vi "test_Multiple Writes and Reads.vi"(8 "error in (no error)":errorcluster, 11 "Scalar Channels Testing in":refnum<class "FPGA Addon Scalar Channels System Tests.lvclass">) -> (0 "error out":errorcluster, 3 "Scalar Channels Testing out":refnum<class "FPGA Addon Scalar Channels System Tests.lvclass">)   [LabVIEW 2018, in "FPGA Addon Scalar Channels System Tests.lvclass"]
uses:
  FPGA Addon Scalar Channels System Tests.lvclass
  C:/Dev/niveristand-fpga-addon-custom-device-1/Source/Tests/FPGA Addon Test Class/FPGA Addon Test Class.lvclass
  C:/Program Files (x86)/National Instruments/LabVIEW 2018/vi.lib/NI/NI VS CD Testing Tools/VeriStandTestCase/VeriStandTestCase.lvclass
  FPGA Addon Test Class/FPGA Addon Test Class.lvclass/FPGA Addon Test Class.ctl
  FPGA Addon Test Class/FPGA Addon Test Class.lvclass
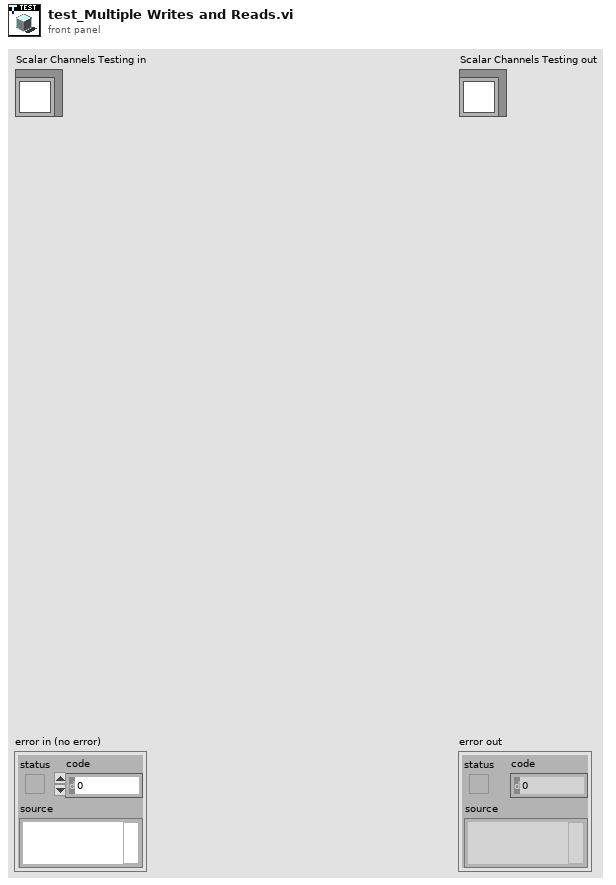
[diagram p1: front panel]
types:
  T1 = typedef "NI_VS Workspace ExecutionAPI.lvlib/WorkspaceAPI.ctl" = refnum<k24>
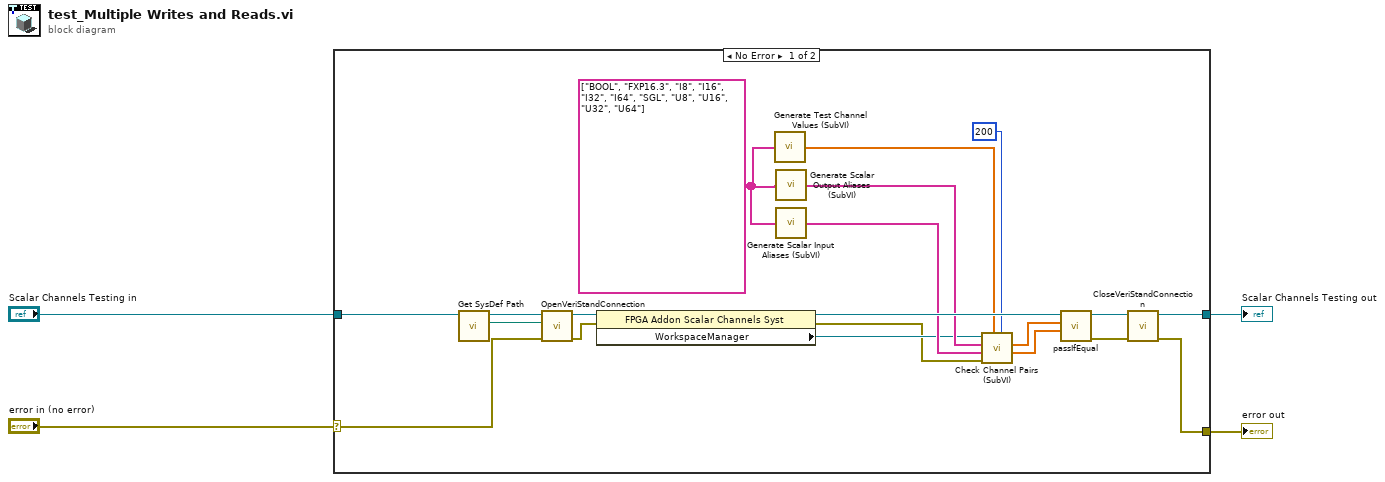
[diagram p0: block diagram]
diagram:
  n1 = case shown="No Error" "error in (no error)" {
    selector: "error in (no error)" -> [w17 w26]
    tunnel: [w23 w26] -> w3
    tunnel: [w24 w25] -> w1
    tunnel: "Scalar Channels Testing in" -> [w7 w25]
    frame No Error {
      w12 = string[] ["BOOL", "FXP16.3", "I8", "I16", "I32", "I64", "SGL", "U8", "U16", "U32", "U64"]
      n2 = call "Get SysDef Path.vi"("Scalar Channels Testing in"=w7) -> ("SysDef Path"=w5:path, "Scalar Channels Testing out"=w6:refnum<class "FPGA Addon Scalar Channels System Tests.lvclass">)  [unwired: 9 in]
      n3 = call-dynamic "OpenVeriStandConnection.vi"("error in (no error)"=w17, "System Definition File"=w5, "VeriStand Test Case in"=w6) -> ("error out"=w22:errorcluster, "VeriStand Test Case out"=w21:refnum<class "FPGA Addon Scalar Channels System Tests.lvclass">)  [unwired: 6 in, 1 out]
      n4 = property class="FPGA Addon Scalar Channels Syst"(reference=w21, error in=w22) -> (reference out=w19:refnum<class "FPGA Addon Scalar Channels System Tests.lvclass">, error out=w8:errorcluster, "WorkspaceManager"=w9:T1)
      n5 = call "Generate Test Channel Values (SubVI).vi"("Aliases in"=w12) -> ("Test Channel Values out"=w14:dbl[])
      n6 = call "Generate Scalar Output Aliases (SubVI).vi"("Aliases Seed"=w12) -> ("Scalar Output Aliases"=w11:string[])
      n7 = call "Generate Scalar Input Aliases (SubVI).vi"("Aliases Seed"=w12) -> ("Scalar Input Aliases"=w10:string[])
      n8 = call "Check Channel Pairs (SubVI).vi"("milliseconds to wait"=u32 200, "Test Values"=w14, "error in (no error)"=w8, "Scalar Input Aliases"=w10, "Scalar Output Aliases"=w11, ".NET Refnum in"=w9) -> ("Input Scalar Channel Values"=w15:dbl[], "Output Scalar Channel Values"=w16:dbl[])  [unwired: 2 in, 2 out]
      n9 = call-dynamic "passIfEqual.vi"("y"=w15, "x"=w16, "TestCase in"=w19) -> ("error out"=w20:errorcluster, "TestCase out"=w18:refnum<class "FPGA Addon Scalar Channels System Tests.lvclass">)  [unwired: 7 in]
      n10 = call-dynamic "CloseVeriStandConnection.vi"("error in (no error)"=w20, "VeriStand Test Case in"=w18) -> ("error out"=w23:errorcluster, "VeriStand Test Case out"=w24:refnum<class "FPGA Addon Scalar Channels System Tests.lvclass">)  [unwired: 8 in]
    }
    frame Error {
    }
  }
  "error out" <- w3
  "Scalar Channels Testing out" <- w1
